vi "index_around_me.vi"(10 "my position":i32[](array[numeric]), 11 "board_size":i32[](array[numeric])) -> (3 "index_out":cluster{"Numeric":i32, "Numeric":i32}[](array[cluster]))   [LabVIEW 2020, in "The_Hill_Youth.lvlib" / "MySquare.lvclass"]
uses:
  MySquare.lvclass
  SquareBattle/Direction.ctl
  SquareBattle/SquareBattle.lvlib
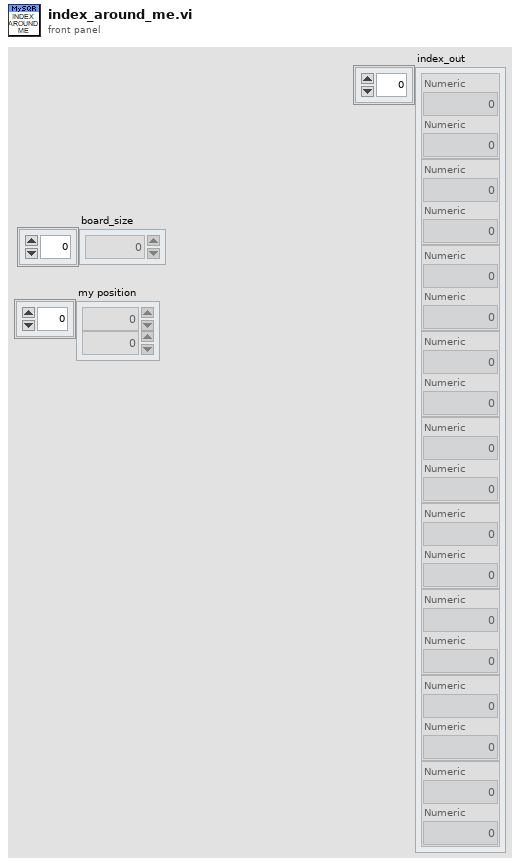
[diagram p1: front panel]
types:
  T1 = typedef "SquareBattle.lvlib/Direction.ctl" = enum16{"NW", "N", "NE", "E", "SE", "S", "SW", "W"}
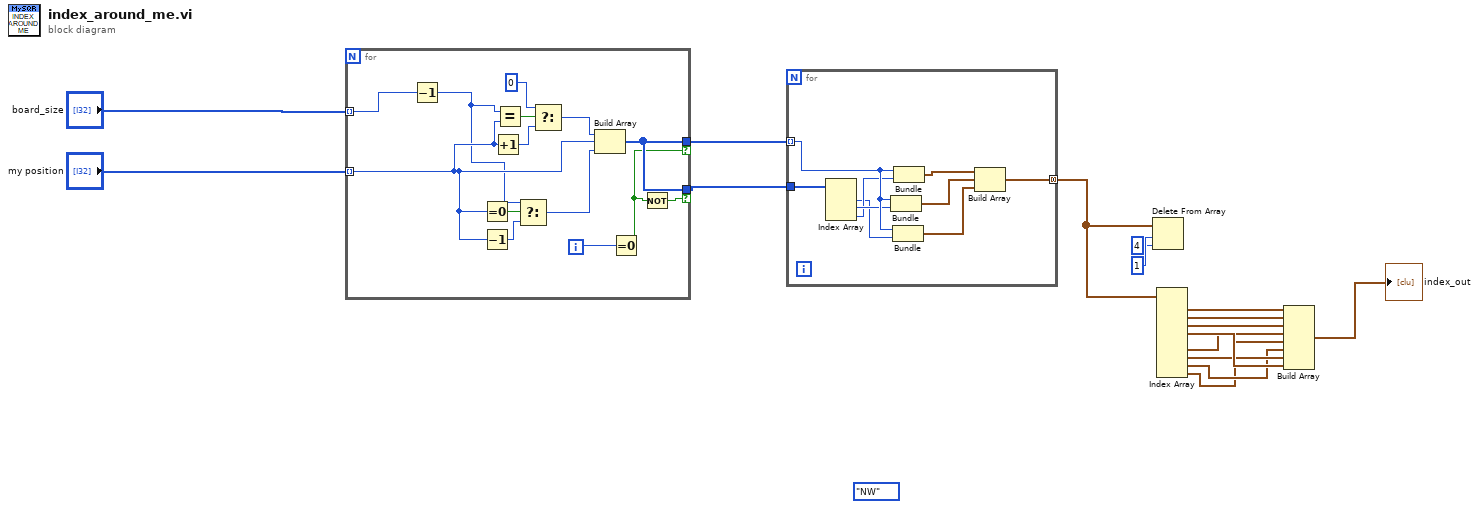
[diagram p0: block diagram]
diagram:
  (unwired) Direction."NW" ("Direction")
  n1 = for {
    tunnel: "board_size" -> [w18] mode=indexing
    tunnel: "my position" -> [w23] mode=indexing
    tunnel: [w22] -> w2 if=w20
    tunnel: [w22] -> w1 if=w19
    i -> [w21]
    n2 = Decrement(x=w18) -> (x-1=w17:i32)
    n3 = Equal To 0?(x=w23) -> (x = 0?=w30:bool)
    n4 = Decrement(x=w23) -> (x-1=w29:i32)
    n5 = Increment(x=w23) -> (x+1=w27:i32)
    n6 = Equal?(x=w17, y=w23) -> (x = y?=w28:bool)
    n7 = Select(t=w17, s=w30, f=w29) -> (s? t:f=w25:i32)
    n8 = Select(t=0, s=w28, f=w27) -> (s? t:f=w24:i32)
    n9 = Build Array(w24, w23, w25) -> (w22:i32[])
    n10 = Equal To 0?(x=w21) -> (x = 0?=w20:bool)
    n11 = Not(x=w20) -> (.not. x?=w19:bool)
  }
  n12 = for {
    tunnel: w2 -> [w38] mode=indexing
    tunnel: w1 -> [w39]
    tunnel: [w33] -> w10 mode=concatenating
    n13 = Index Array(array=w39) -> (element #1=w31:i32, element #2=w37:i32, element #3=w32:i32)  [unwired: 3 in]
    n14 = Bundle("Numeric"=w38, "Numeric"=w37) -> (w35:cluster{"Numeric":i32, "Numeric":i32})  [unwired: 1 in]
    n15 = Bundle("Numeric"=w38, "Numeric"=w31) -> (w34:cluster{"Numeric":i32, "Numeric":i32})  [unwired: 1 in]
    n16 = Bundle("Numeric"=w38, "Numeric"=w32) -> (w36:cluster{"Numeric":i32, "Numeric":i32})  [unwired: 1 in]
    n17 = Build Array(w36, w35, w34) -> (w33:cluster{"Numeric":i32, "Numeric":i32}[])
  }
  n18 = Delete From Array(array=w10, length=1, index=4) -> ()  [unwired: 2 out]
  n19 = Index Array(array=w10) -> (element #1=w7:cluster{"Numeric":i32, "Numeric":i32}, element #2=w8:cluster{"Numeric":i32, "Numeric":i32}, element #3=w9:cluster{"Numeric":i32, "Numeric":i32}, element #4=w16:cluster{"Numeric":i32, "Numeric":i32}, element #6=w15:cluster{"Numeric":i32, "Numeric":i32}, element #7=w13:cluster{"Numeric":i32, "Numeric":i32}, element #8=w12:cluster{"Numeric":i32, "Numeric":i32}, element #9=w11:cluster{"Numeric":i32, "Numeric":i32})  [unwired: 9 in, 1 out]
  n20 = Build Array(w7, w8, w9, w15, w11, w12, w13, w16) -> (→"index_out":cluster{"Numeric":i32, "Numeric":i32}[])
